vi "Kopia HSOpMux.vi"() -> ()   [LabVIEW 2013]
uses:
  Multiplexer_Opmux.lvclass
  HS3.llb/GetDataVoltCh_ForGraphs.vi
  OverallRoutines/HS3OverallRoutines.lvlib
panel:
  in  "Run":bool
  out "Channels":refnum<vi>[](array[refnum])
  out "Ch8":dbl[](graph)
  out "Ch7":dbl[](graph)
  out "Ch6":dbl[](graph)
  out "Ch5":dbl[](graph)
  out "Ch4":dbl[](graph)
  out "Ch3":dbl[](graph)
  out "Ch2":dbl[](graph)
  out "Ch1":dbl[](graph)
  in  "Scan":bool
  in  "Set":bool
  in  "Length":dbl=1.0 caption="Length (us)" min=0.1 max=6.3 step=0.1
  in  "Voltage":dbl min=0.0 max=1023.0 step=1.0
  in  "Into":u16[](array[numeric])
  in  "Forward":u16[](array[numeric])
  in  "Signal Frequency":u32(ring)=10000000 items=["5Mhz"=5000000, "10Mhz"=10000000, "25Mhz"=25000000]
  in  "Shutdown":bool
  out "Acq":bool caption="Acquiring"
  out "SampleFrequency":dbl format="%#_8g"
  out "ChArray":dbl[](array[numeric])
  out "Serial":i32
  out "DllPath":path
  out "HandyScope":bool
  out "Multiplexer":bool
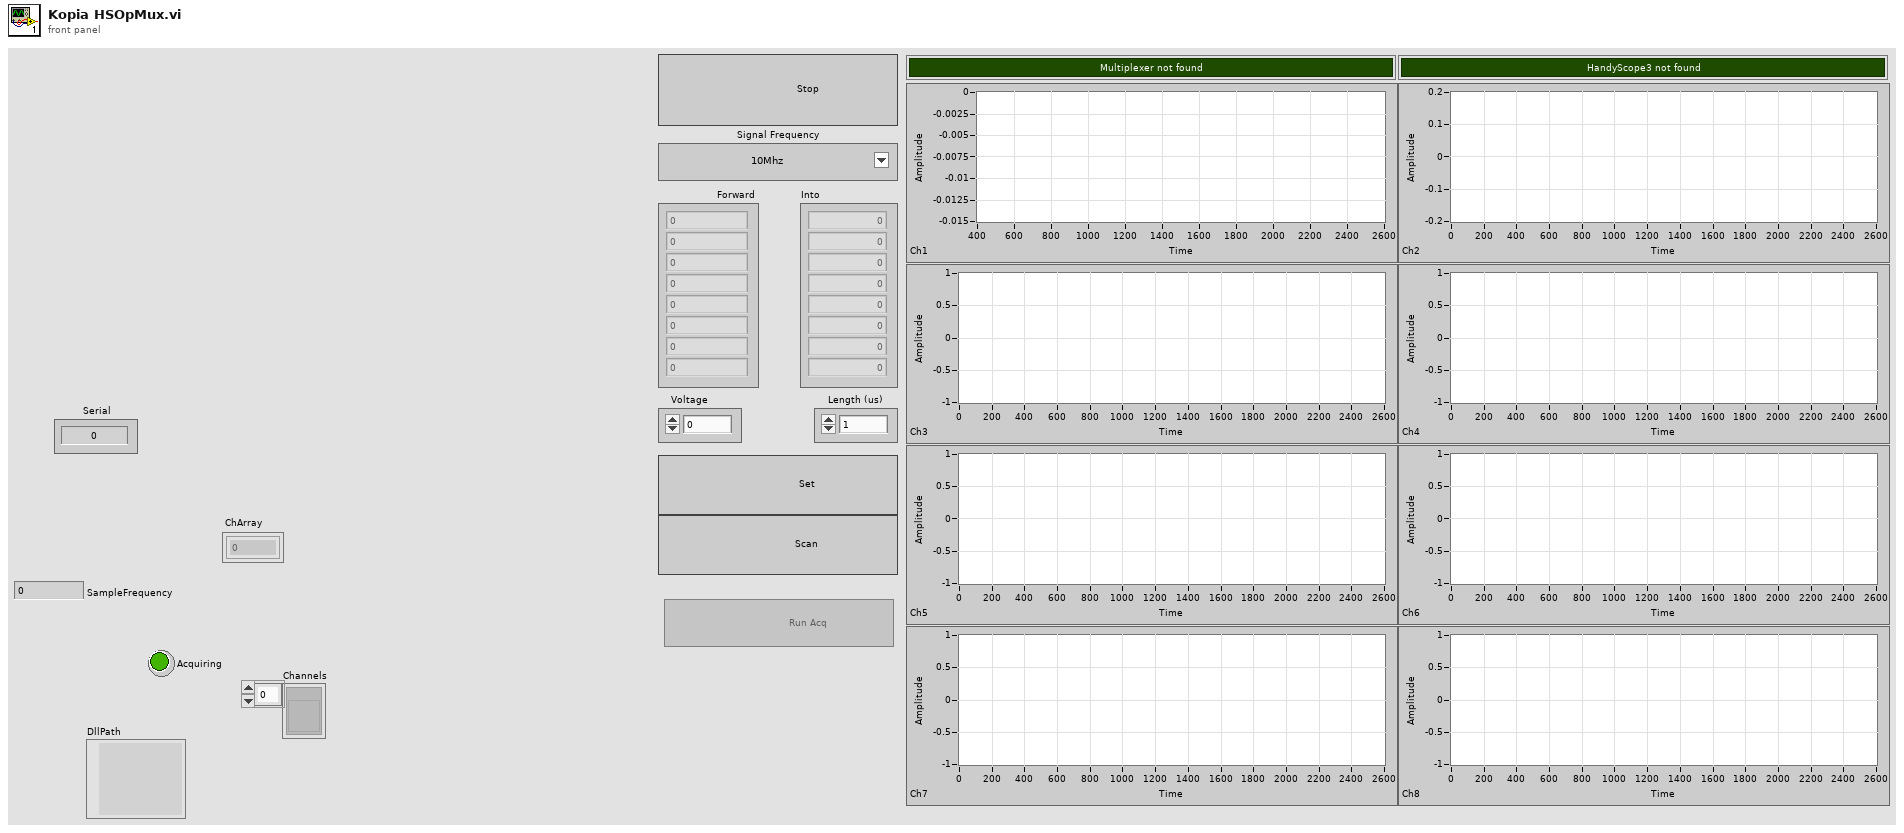
[diagram p1: front panel]
types:
  T1 = cluster{"trgSource":u16, "trgMode":u16, "trgLevel":dbl}
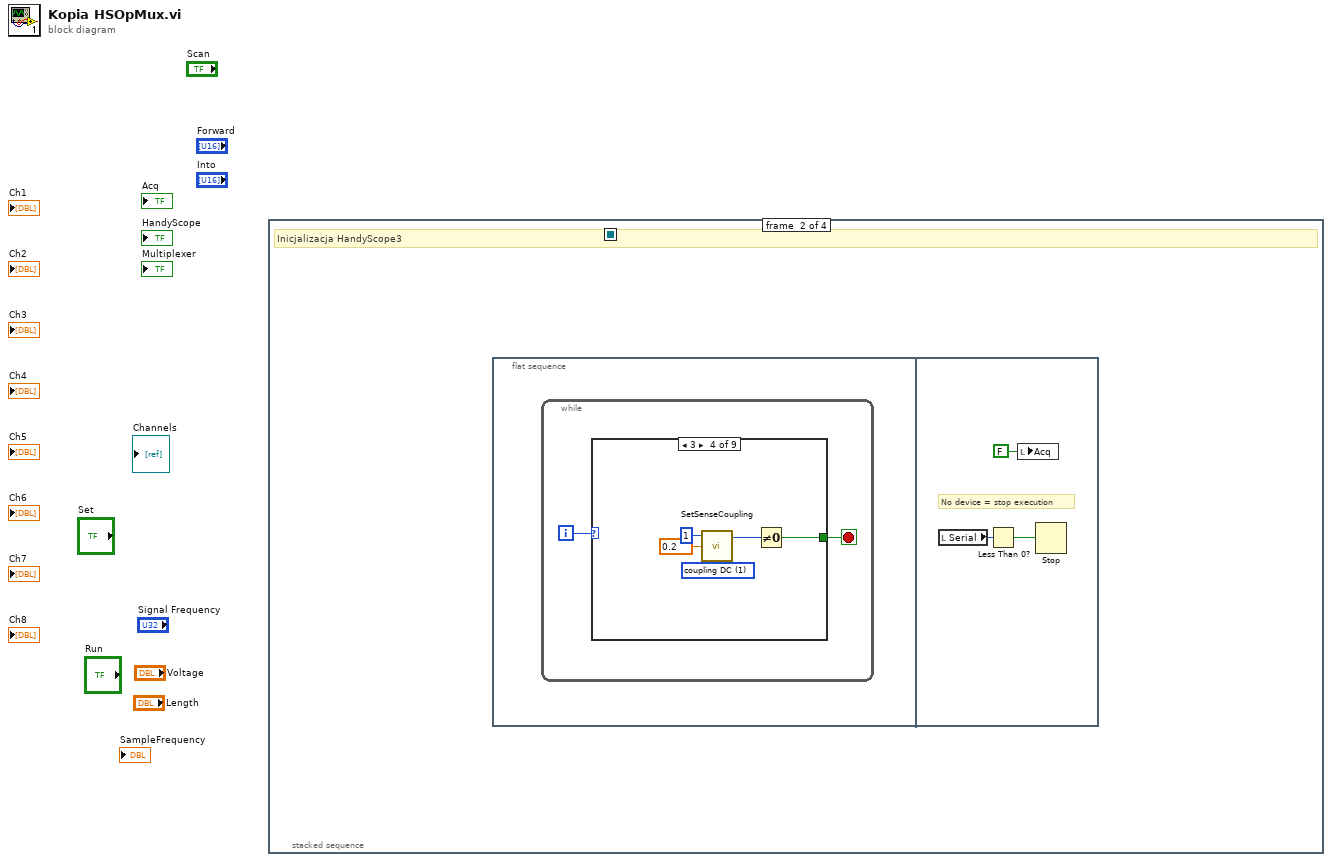
[diagram p0: block diagram]
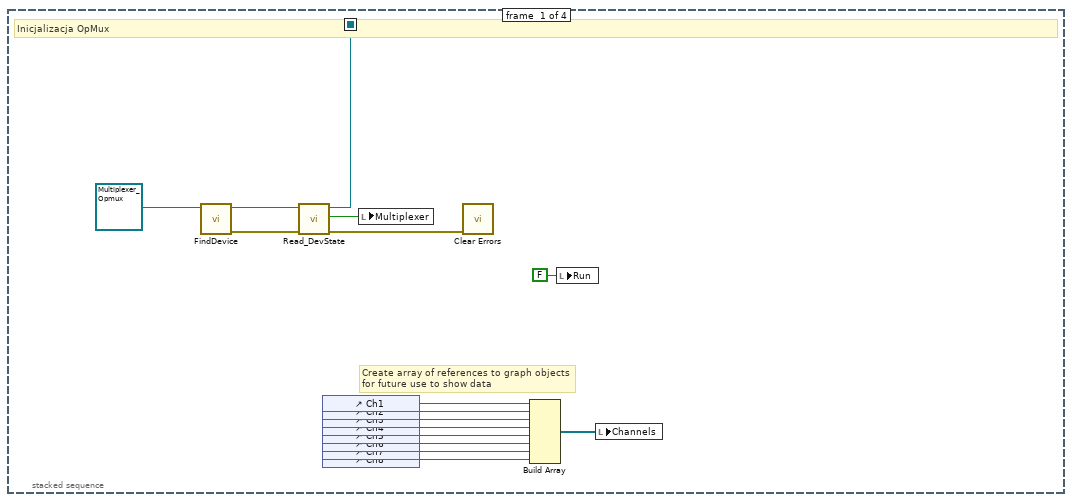
[diagram p2: hidden frame]
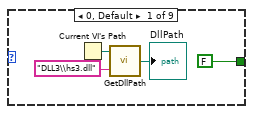
[diagram p3: hidden frame]
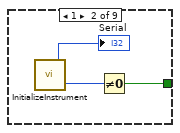
[diagram p4: hidden frame]
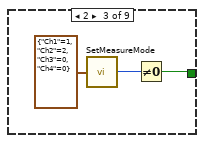
[diagram p5: hidden frame]
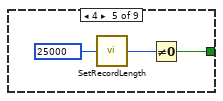
[diagram p6: hidden frame]
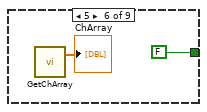
[diagram p7: hidden frame]
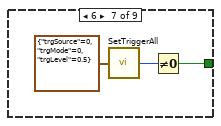
[diagram p8: hidden frame]
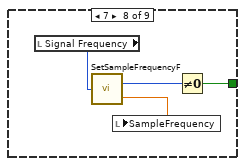
[diagram p9: hidden frame]
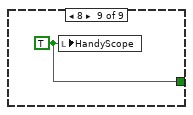
[diagram p10: hidden frame]
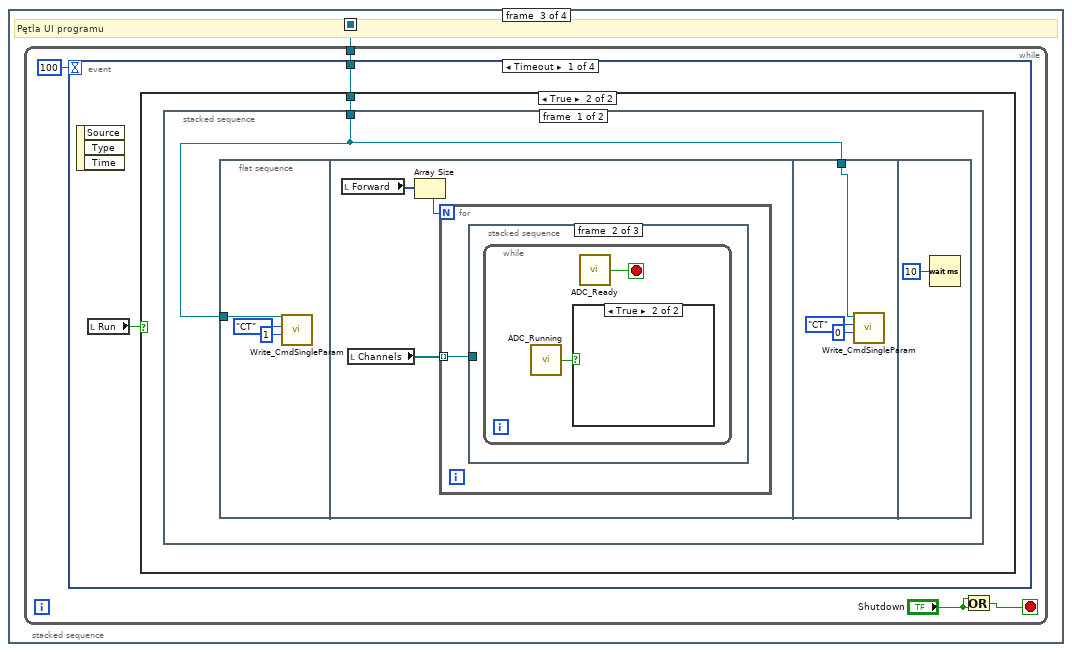
[diagram p11: hidden frame]
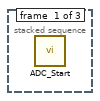
[diagram p13: hidden frame]
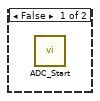
[diagram p14: hidden frame]
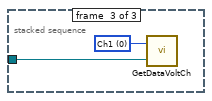
[diagram p15: hidden frame]
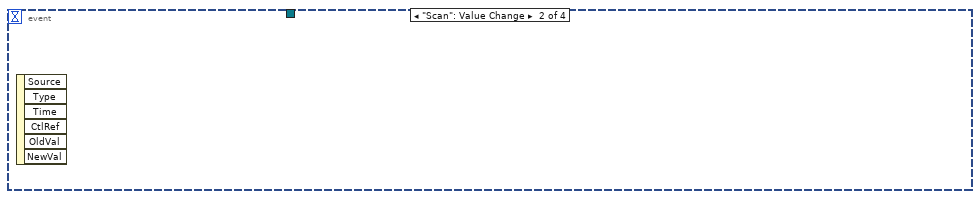
[diagram p17: hidden frame]
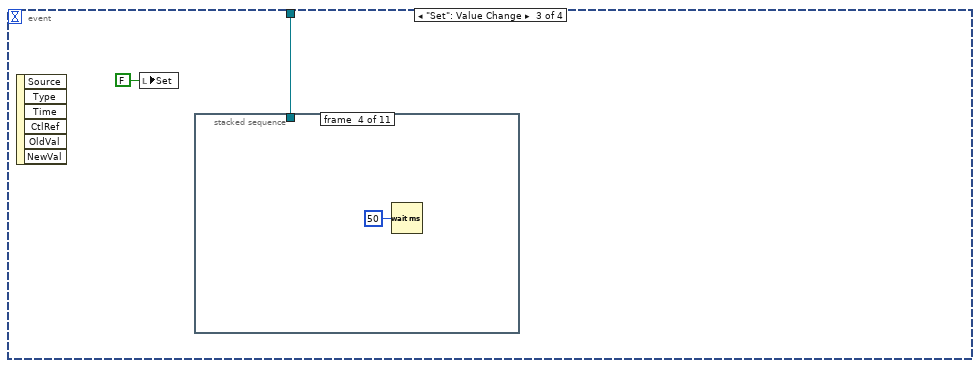
[diagram p18: hidden frame]
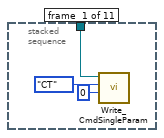
[diagram p19: hidden frame]
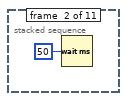
[diagram p20: hidden frame]
diagram:
  n1 = stacked-sequence {
    seq-local: [w13 _ _ _] -> [_ _ w50 _]
    frame #0 {
      # "Create array of references to graph objects\nfor future use to show data"
      # "Inicjalizacja OpMux"
      n2 = call-dynamic "FindDevice.vi"("Multiplexer_Opmux in"=refnum<class "Multiplexer_Opmux.lvclass"> refnum) -> ("error out"=w12:errorcluster, "Multiplexer_Opmux out"=w15:refnum<class "Multiplexer_Opmux.lvclass">)  [unwired: 8 in, 1 out]
      n3 = call-dynamic "Read_DevState.vi"("error in (no error)"=w12, "Multiplexer_Opmux in"=w15) -> ("error out"=w11:errorcluster, "DevState"=w14:bool, "Multiplexer_Opmux out"=w13:refnum<class "Multiplexer_Opmux.lvclass">)  [unwired: 7 in]
      n4 = control-ref of="Ch1"() -> (w10:refnum<vi>)
      n5 = control-ref of="Ch2"() -> (w9:refnum<vi>)
      n6 = control-ref of="Ch3"() -> (w8:refnum<vi>)
      n7 = control-ref of="Ch4"() -> (w7:refnum<vi>)
      n8 = control-ref of="Ch5"() -> (w6:refnum<vi>)
      n9 = control-ref of="Ch6"() -> (w5:refnum<vi>)
      n10 = control-ref of="Ch7"() -> (w4:refnum<vi>)
      n11 = control-ref of="Ch8"() -> (w3:refnum<vi>)
      n12 = local write "Multiplexer"(w14) -> ()
      n13 = call <vilib>:"Clear Errors.vi"("error in (no error)"=w11) -> ()  [unwired: 6 in, 1 out]
      n14 = Build Array(w10, w9, w8, w7, w6, w5, w4, w3) -> (w2:refnum<vi>[])
      n15 = local write "Run"(FALSE ("Run")) -> ()
      n16 = local write "Channels"(w2) -> ()
    }
    frame #1 {
      # "Inicjalizacja HandyScope3"
      n17 = flat-sequence {
        frame #0 {
          n18 = while {
            i -> [w18]
            stop <- w17 stop-if-true
            n19 = case shown="3" w18 {
              tunnel: [FALSE w23 w27 w29 w35 FALSE w40 w45 w46] -> w17
              frame 0, Default {
                n20 = Current VI's Path() -> (path=w20:path)
                n21 = call "GetDllPath.vi"("DllName"="DLL3\\hs3.dll", "path"=w20) -> ("DllPath"=→"DllPath":path)
              }
              frame 1 {
                n22 = call "InitializeInstrument.vi"() -> ("ErrorCode"=w24:i16, "Serial"=→"Serial":i32)
                n23 = Not Equal To 0?(x=w24) -> (x != 0?=w23:bool)
              }
              frame 2 {
                n24 = call "SetMeasureMode.vi"("oModeStack"=cluster{"Ch1":u8, "Ch2":u8, "Ch3":u8, "Ch4":u8} {"Ch1"=1, "Ch2"=2, "Ch3"=0, "Ch4"=0}) -> ("ErrorCode"=w26:i16)
                n25 = Not Equal To 0?(x=w26) -> (x != 0?=w27:bool)
              }
              frame 3 {
                w33 = 0.2 items=["0,2"=0.2, "0,8"=0.8, "2"=2.0, "4"=4.0, "20"=20.0, "40"=40.0, "80"=80.0] ("chSense")
                w32 = 1 items=["coupling AC", "coupling DC"] ("chCoupling")
                n26 = call "SetSenseCoupling.vi"("chCoupling"=w32, "chSense"=w33, "chSet"=1) -> ("ErrorCode"=w30:i16)  [unwired: 1 out]
                n27 = Not Equal To 0?(x=w30) -> (x != 0?=w29:bool)
              }
              frame 4 {
                w36 = u32 25000 items=["100"=100, "250"=250, "500"=500, "1000"=1000, "2500"=2500, "5000"=5000, "10000"=10000, "25000"=25000, "50000"=50000, "100000"=100000, "131000"=131000] ("RecordLength")
                n28 = call "SetRecordLength.vi"("RecordLength"=w36) -> ("ErrorCode"=w34:i16)
                n29 = Not Equal To 0?(x=w34) -> (x != 0?=w35:bool)
              }
              frame 5 {
                n30 = call "GetChArray.vi"() -> ("ChArray"=→"ChArray":dbl[])  [unwired: 1 out]
              }
              frame 6 {
                n31 = call "SetTriggerAll.vi"("TriggerSettings"=T1 {"trgSource"=0, "trgMode"=0, "trgLevel"=0.5}) -> ("ErrorCode"=w41:i32)
                n32 = Not Equal To 0?(x=w41) -> (x != 0?=w40:bool)
              }
              frame 7 {
                n33 = local read "Signal Frequency"() -> (w43:u32)
                n34 = call "SetSampleFrequencyF.vi"("Numeric Control"=w43) -> ("ErrorCode"=w44:i16, "oFreq_Set"=w42:dbl)
                n35 = local write "SampleFrequency"(w42) -> ()
                n36 = Not Equal To 0?(x=w44) -> (x != 0?=w45:bool)
              }
              frame 8 {
                w46 = TRUE ("HandyScope")
                n37 = local write "HandyScope"(w46) -> ()
              }
            }
          }
        }
        frame #1 {
          # "No device = stop execution"
          n38 = local read "Serial"() -> (w49:i32)
          n39 = Less Than 0?(x=w49) -> (x < 0?=w48:bool)
          n40 = local write "Acq"(FALSE ("Acq")) -> ()
          n41 = Stop(stop? (T)=w48) -> ()
        }
      }
    }
    frame #2 {
      # "Pętla UI programu"
      n42 = while {
        tunnel: w50 -> [w51]
        stop <- w53 stop-if-true
        n43 = event shown="[0] Timeout" {
          selector: _ -> [_ _ _ _]
          dyn-events: _ -> [_ _ _ _]
          timeout: 100 -> [_ _ _ _]
          tunnel: w51 -> [w56 _ w75 _]
          event Timeout {
            n44 = event-data() -> ()  [unwired: 1 in, 3 out]
            n45 = local read "Run"() -> (w55:bool)
            n46 = case shown="True" w55 {
              tunnel: w56 -> [_ w57]
              frame False {
              }
              frame True {
                n47 = stacked-sequence {
                  tunnel: w57 -> [w58 _]
                  frame #0 {
                    n48 = flat-sequence {
                      tunnel: w58 -> [w61]
                      tunnel: w58 -> [w70]
                      frame #0 {
                        n49 = call-dynamic "Write_CmdSingleParam.vi"("Param"=1, "Command"=enum16{"SA", "GT", "SI", "SL", "ST", "CT"}."CT", "Multiplexer_Opmux in"=w61) -> ()  [unwired: 7 in, 2 out]
                      }
                      frame #1 {
                        n50 = local read "Forward"() -> (w64:u16[])
                        n51 = local read "Channels"() -> (w62:refnum<vi>[])
                        n52 = Array Size(array=w64) -> (size(s)=w63:i32)
                        n53 = for {
                          N: w63 -> [_]
                          tunnel: w62 -> [w65] mode=indexing
                          n54 = stacked-sequence {
                            tunnel: w65 -> [_ _ w68]
                            frame #0 {
                              n55 = call "ADC_Start.vi"() -> ()  [unwired: 1 out]
                            }
                            frame #1 {
                              n56 = while {
                                stop <- w67 stop-if-true
                                n57 = call "ADC_Running.vi"() -> ("Measuring"=w66:bool)
                                n58 = case shown="True" w66 {
                                frame False {
                                n59 = call "ADC_Start.vi"() -> ()  [unwired: 1 out]
                                }
                                frame True {
                                }
                                }
                                n60 = call "ADC_Ready.vi"() -> ("Ready"=w67:bool)
                              }
                            }
                            frame #2 {
                              w69 = u8 0 items=["Ch1", "Ch2", "Ch3", "Ch4"] ("Ch")
                              n61 = call-poly "GetDataVoltCh.vi"("chData"=w68, "Ch"=w69) -> ()  [unwired: 1 out]
                            }
                          }
                        }
                      }
                      frame #2 {
                        n62 = call-dynamic "Write_CmdSingleParam.vi"("Param"=0, "Command"=enum16{"SA", "GT", "SI", "SL", "ST", "CT"}."CT", "Multiplexer_Opmux in"=w70) -> ()  [unwired: 7 in, 2 out]
                      }
                      frame #3 {
                        n63 = Wait (ms)(milliseconds to wait=u32 10) -> ()  [unwired: 1 out]
                      }
                    }
                  }
                  frame #1 {
                  }
                }
              }
            }
          }
          event "Scan": Value Change {
            n64 = event-data() -> ()  [unwired: 1 in, 6 out]
          }
          event "Set": Value Change {
            n65 = event-data() -> ()  [unwired: 1 in, 6 out]
            n66 = local write "Set"(FALSE ("Set")) -> ()
            n67 = stacked-sequence {
              tunnel: w75 -> [w78 _ w80 _ w85 _ w91 _ w95 _ _]
              frame #0 {
                n68 = call-dynamic "Write_CmdSingleParam.vi"("Param"=0, "Command"=enum16{"SA", "GT", "SI", "SL", "ST", "CT"}."CT", "Multiplexer_Opmux in"=w78) -> ()  [unwired: 7 in, 2 out]
              }
              frame #1 {
                n69 = Wait (ms)(milliseconds to wait=u32 50) -> ()  [unwired: 1 out]
              }
              frame #2 {
                n70 = local read "Forward"() -> (w83:u16[])
                n71 = local read "Into"() -> (w82:u16[])
                n72 = call-dynamic "Write_CmdMultipleParam.vi"("Command"=enum16{"ST"}."ST", "Table2"=w82, "Table1"=w83, "Multiplexer_Opmux in"=w80) -> ()  [unwired: 6 in, 2 out]
              }
              frame #3 {
                n73 = Wait (ms)(milliseconds to wait=u32 50) -> ()  [unwired: 1 out]
              }
              frame #4 {
                n74 = local read "Length"() -> (w87:dbl)
                n75 = Multiply(x=w87, y=10.0) -> (x*y=w88:dbl)
                n76 = call-dynamic "Write_CmdSingleParam.vi"("Param"=w88, "Command"=enum16{"SA", "GT", "SI", "SL", "ST", "CT"}."SL", "Multiplexer_Opmux in"=w85) -> ()  [unwired: 7 in, 2 out]
              }
              frame #5 {
                n77 = Wait (ms)(milliseconds to wait=u32 50) -> ()  [unwired: 1 out]
              }
              frame #6 {
                n78 = local read "Voltage"() -> (w93:dbl)
                n79 = call-dynamic "Write_CmdSingleParam.vi"("Param"=w93, "Command"=enum16{"SA", "GT", "SI", "SL", "ST", "CT"}."SI", "Multiplexer_Opmux in"=w91) -> ()  [unwired: 7 in, 2 out]
              }
              frame #7 {
                n80 = Wait (ms)(milliseconds to wait=u32 50) -> ()  [unwired: 1 out]
              }
              frame #8 {
                n81 = call-dynamic "Buffer_flushBuffer.vi"("Multiplexer_Opmux in"=w95) -> ()  [unwired: 9 in, 2 out]
              }
              frame #9 {
                n82 = Wait (ms)(milliseconds to wait=u32 25) -> ()  [unwired: 1 out]
              }
              frame #10 {
                n83 = local write "Run"(TRUE ("Run")) -> ()
              }
            }
          }
          event "Signal Frequency": Value Change {
            n84 = event-data() -> ("NewVal"=w98:u32)  [unwired: 1 in, 5 out]
            n85 = stacked-sequence {
              tunnel: w98 -> [w104 _]
              frame #0 {
                # "Do 100us sygnał zmieniamy automatycznie"
                n86 = call "SetSampleFrequencyF.vi"("Numeric Control"=w104) -> ("ErrorCode"=w103:i16, "oFreq_Set"=w102:dbl)
                n87 = local write "SampleFrequency"(w102) -> ()
                n88 = Multiply(x=w102, y=0.0001) -> (x*y=w100:dbl)
                n89 = To Unsigned Long Integer(number=w100) -> (unsigned 32bit integer=w101:u32)
                n90 = call "Error Converter (ErrCode or Status).vi"("error code"=w103) -> ()  [unwired: 10 in, 1 out]
                n91 = call "SetRecordLength.vi"("RecordLength"=w101) -> ()  [unwired: 1 out]
              }
              frame #1 {
              }
            }
          }
        }
        n92 = Or(x="Shutdown", y="Shutdown") -> (x .or. y?=w53:bool)
      }
    }
    frame #3 {
      # "Rozłączenie urządzeń po zakończeniu działania programu"
    }
  }
